vi "Set Async Status.vi"(7 "State":T1, 8 "error in (no error)":errorcluster, 11 "queue in":refnum<queue>) -> (0 "error out":errorcluster, 3 "queue out":refnum<queue>)   [LabVIEW 2011, in "Switch-DMM Custom Device.lvlib"]
uses:
  Switch-DMM Custom Device.lvlib
  Controls/Async State.ctl
  Controls/Async Status.ctl
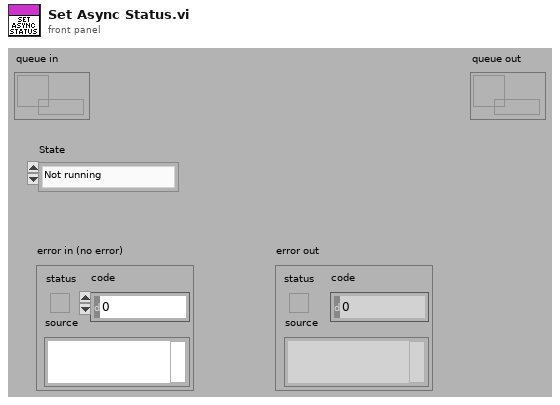
[diagram p1: front panel]
types:
  T1 = typedef "Switch-DMM Custom Device.lvlib/Async State.ctl" = enum16{"Not running", "Initializing", "Waiting on start cmd", "Running", "Stopped"}
  T2 = typedef "Switch-DMM Custom Device.lvlib/Async Status.ctl" = cluster{"State":T1, "error":errorcluster}
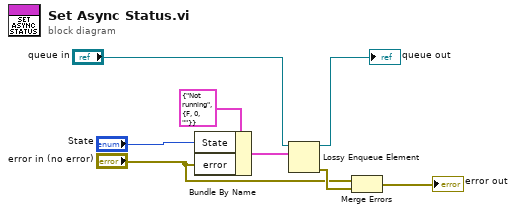
[diagram p0: block diagram]
diagram:
  n1 = Bundle By Name(cluster=T2 {"State"=enum."Not running", "error"={"status"=FALSE, "code"=0, "source"=""}} ("Async Status"), "State"="State", "error"="error in (no error)") -> (w6:T2)
  n2 = Lossy Enqueue Element(queue="queue in", element=w6) -> (queue out=→"queue out":refnum<queue>, error out=w5:errorcluster)  [unwired: 1 in, 2 out]
  n3 = Merge Errors("error in (no error)", w5) -> (→"error out":errorcluster)
